vi "ma_Tone estimation subroutine G(f) (first derivative).vi"   [LabVIEW 2020, in "NI_MAPro.lvlib"]
uses:
  NI_MAPro.lvlib
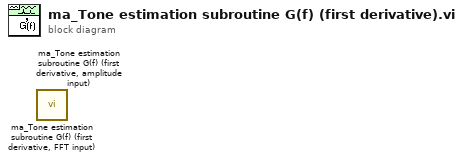
[diagram p0: block diagram]
diagram:
  n1 = call "ma_Tone estimation subroutine G(f) (first derivative, FFT input).vi"() -> ()  [unwired: 4 in, 1 out]
  n2 = call "ma_Tone estimation subroutine G(f) (first derivative, amplitude input).vi"() -> ()  [unwired: 4 in, 1 out]
